vi "Clear.vi"(8 "error in (no error)":errorcluster, 11 "VISA Resource Name":refnum<visa-resource-name>) -> (0 "error out":errorcluster, 3 "VISA Resource Name Out":refnum<visa-resource-name>)   [LabVIEW 2010, in "Tektronix TDS 3000 Series.lvlib"]
doc: "Chooses the correct method and clears the buffer of the instrument.\n\nNotes:\n\n(1) If timeouts are happening frequently and the I/O port being used is serial, try increasing the delay time after the VISA clear for the instrument to catch up and get back to the ready state before the next command is sent."
uses:
  <instrlib>/Tektronix TDS 3000 Series/Tektronix TDS 3000 Series.lvlib
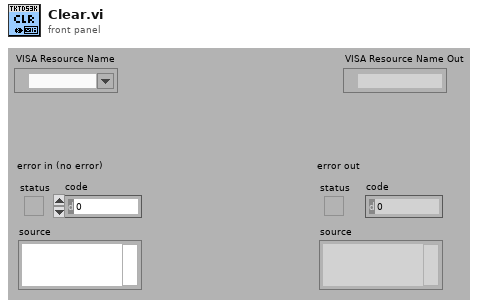
[diagram p1: front panel]
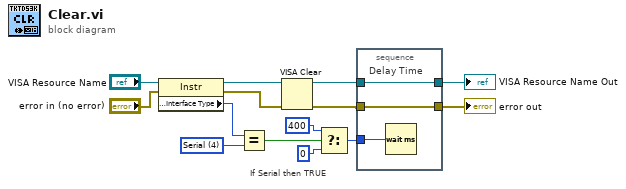
[diagram p0: block diagram]
diagram:
  w6 = u16 4 items=["GPIB"=1, "VXI"=2, "GPIB-VXI"=3, "Serial"=4, "PXI"=5, "TCPIP"=6, "USB"=7] ("Interface Information:Interface Type")
  # "If Serial then TRUE"
  n1 = property class="Instr"(reference="VISA Resource Name", error in="error in (no error)") -> (reference out=w3:refnum<visa-resource-name>, error out=w2:errorcluster, "Interface Information:Interface Type"=w7:u16)
  n2 = Equal?(x=w7, y=w6) -> (x = y?=w1:bool)
  n3 = VISA Clear(VISA resource name=w3, error in (no error)=w2) -> (VISA resource name out=w11:refnum<visa-resource-name>, error out=w10:errorcluster)
  n4 = Select(t=u32 400, s=w1, f=u32 0 ("t")) -> (s? t:f=w12:u32)
  n5 = stacked-sequence {
    tunnel: w11 -> [w17]
    tunnel: [w17] -> w9
    tunnel: w10 -> [w16]
    tunnel: [w16] -> w8
    tunnel: w12 -> [w15]
    frame #0 {
      # "Delay Time"
      n6 = Wait (ms)(milliseconds to wait=w15) -> ()  [unwired: 1 out]
    }
  }
  "error out" <- w8
  "VISA Resource Name Out" <- w9
